vi "AutoSystem.vi"() -> ()   [LabVIEW 2025]
panel:
  out "Function":string
  out "Parm 2":dbl format="%11.2f"
  out "Parm 1":dbl format="%11.2f"
  out "Time out Sec":dbl format="%11.2f"
  out "Parm 3":dbl format="%11.2f"
  out "Cmd":dbl format="%13.0f"
  # "AUTO"
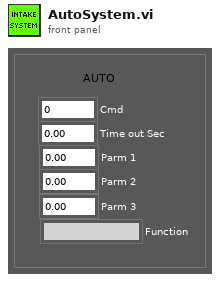
[diagram p1: front panel]
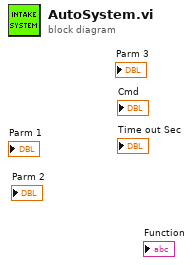
[diagram p0: block diagram]
diagram:
